vi "name.vi"(9 "Time":bool, 10 "Date":bool, 11 "initial string":string) -> (3 "initial string 2":string)   [LabVIEW 2014]
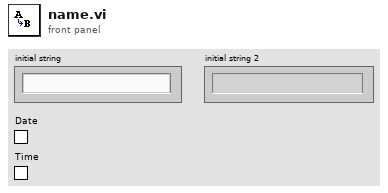
[diagram p1: front panel]
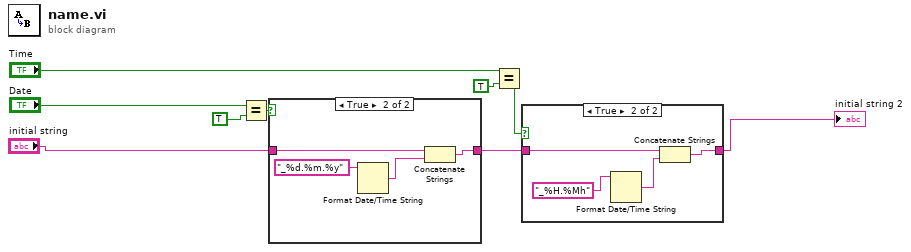
[diagram p0: block diagram]
diagram:
  n1 = Equal?(x="Date", y=TRUE) -> (x = y?=w8:bool)
  n2 = case shown="True" w8 {
    tunnel: [w10 w13] -> w5
    tunnel: "initial string" -> [w10 w11]
    frame False {
    }
    frame True {
      n3 = Format Date/Time String(time format string (%c)="_%d.%m.%y") -> (date/time string=w12:string)  [unwired: 2 in]
      n4 = Concatenate Strings(w11, w12) -> (w13:string)
    }
  }
  n5 = Equal?(x="Time", y=TRUE) -> (x = y?=w6:bool)
  n6 = case shown="True" w6 {
    tunnel: w5 -> [w15 w17]
    tunnel: [w15 w19] -> w1
    frame False {
    }
    frame True {
      n7 = Format Date/Time String(time format string (%c)="_%H.%Mh") -> (date/time string=w16:string)  [unwired: 2 in]
      n8 = Concatenate Strings(w17, w16) -> (w19:string)
    }
  }
  "initial string 2" <- w1
